vi "XML Script - Flat Sequence Frame.vi"(2 "out":i32=-1, 4 "diagram (XML)":string, 6 "name":string, 9 "prefix (name)":string, 10 "in":i32=-1) -> (5 "name (wire source)":string, 7 "XML Script Command - Flat Sequence Frame":string)   [LabVIEW 2020]
uses:
  <vilib>/_script/XML Scripting/XML Script Tag.ctl
  <vilib>/_script/XML Scripting/XML Script Attribute.ctl
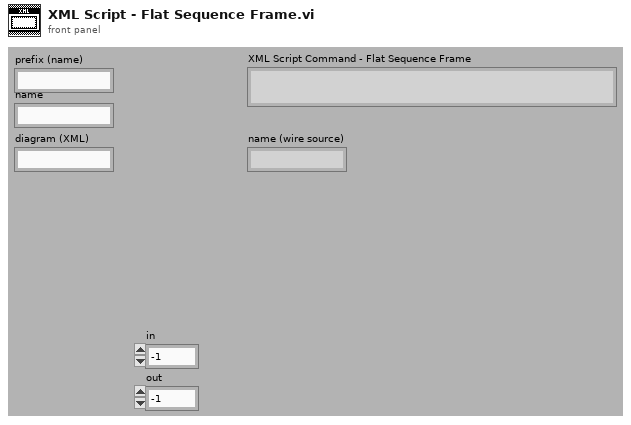
[diagram p1: front panel]
types:
  T1 = typedef "XML Script Attribute.ctl" = enum16{"name", "style", "path", "position", "in", "out", "width", "height", "index", "value", "default", "location", "offset", "typeindex", "size", "source", "destination", "indicator", "type", "controlname", "label", "conpaneidx", "mode", "description", "hasCondTerm", "linkIdentity", "caseselectortype", "concatInputs", "inName", "instantiationpath", "loopCondition", "IndexMode", "formulaInputs", "formulaOutputs", "msnFuncName", "msnIsDynamic", "msnIsODEUserFunction", "ignoreSearchDialog"}
  T2 = typedef "XML Script Tag.ctl" = enum16{"Script", "Function", "SubVI", "GrowableFunction", "Structure", "MultiframeStructure", "Frame", "Tunnel", "ShiftRegister", "Constant", "Control", "Terminal", "Wire", "StaticVIReference", "ControlTerminal", "CompoundArithmetic", "FlatSequence", "FlatSequenceFrame", "MathScriptCallByRef", "BuildArray", "GenericSubVI", "MathScriptNode"}
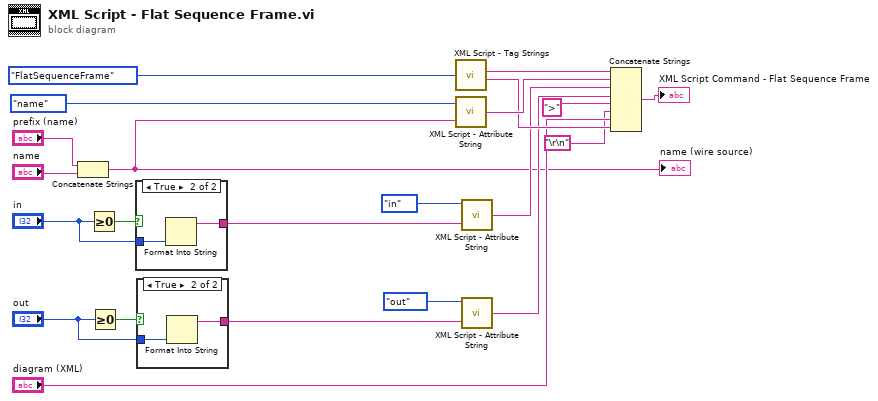
[diagram p0: block diagram]
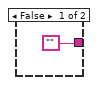
[diagram p2: hidden frame]
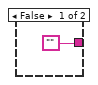
[diagram p3: hidden frame]
diagram:
  n1 = Concatenate Strings("prefix (name)", "name") -> (w1:string)
  "name (wire source)" <- w1
  n2 = Greater Or Equal To 0?(x="in") -> (x >= 0?=w8:bool)
  n3 = Greater Or Equal To 0?(x="out") -> (x >= 0?=w11:bool)
  n4 = case shown="True" w8 {
    tunnel: "in" -> [_ w25]
    tunnel: ["" w24] -> w10
    frame False {
    }
    frame True {
      n5 = Format Into String(w25) -> (resulting string=w24:string)  [unwired: 3 in, 1 out]
    }
  }
  n6 = case shown="True" w11 {
    tunnel: "out" -> [_ w28]
    tunnel: ["" w27] -> w13
    frame False {
    }
    frame True {
      n7 = Format Into String(w28) -> (resulting string=w27:string)  [unwired: 3 in, 1 out]
    }
  }
  n8 = call <vilib>:"XML Script - Tag Strings.vi"("XML Script Tag"=XML_Script_Tag."FlatSequenceFrame") -> ("XML String - Begin Tag"=w21:string, "XML String - End Tag"=w17:string)  [unwired: 2 in]
  n9 = call <vilib>:"XML Script - Attribute String.vi"("Attribute String"=w1, "XML Script Attribute"=XML_Script_Attribute."name") -> ("XML Script - Attribute String"=w18:string)
  n10 = call <vilib>:"XML Script - Attribute String.vi"("Attribute String"=w10, "XML Script Attribute"=XML_Script_Attribute."in") -> ("XML Script - Attribute String"=w5:string)
  n11 = call <vilib>:"XML Script - Attribute String.vi"("Attribute String"=w13, "XML Script Attribute"=XML_Script_Attribute."out") -> ("XML Script - Attribute String"=w6:string)
  n12 = Concatenate Strings(w21, w18, w5, w6, ">" ("string"), "\r\n", "diagram (XML)", w17) -> (→"XML Script Command - Flat Sequence Frame":string)
